vi "CheckAcqErrTlog.vi"(4 "error in":errorcluster) -> (0 "error out":errorcluster, 2 "Erreur":bool)   [LabVIEW 2010]
doc: "Ce Vi prend un tableau de donnée et convertit chaque donées selon la fonction spécifié par l'indicateur du même index dans la table de conversion."
uses:
  <userlib>/TLogger/AcqErrorGlobalTlog.vi
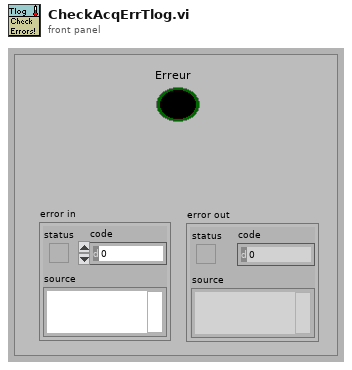
[diagram p1: front panel]
types:
  T1 = enum32{"Invalid", "Standard", "Closed", "Hidden", "Minimized", "Maximized"}
  T2 = enum32{"Bad", "Idle", "Run top level", "Running"}
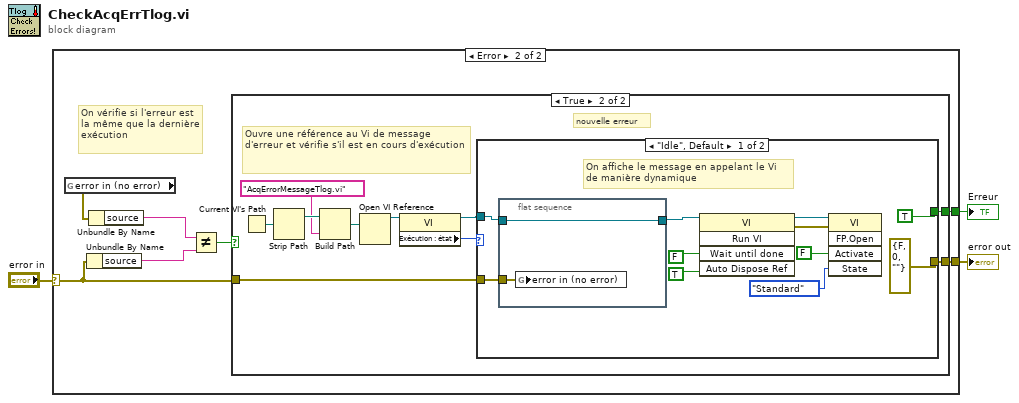
[diagram p0: block diagram]
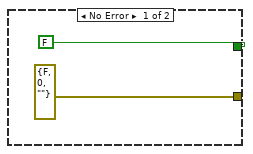
[diagram p2: hidden frame]
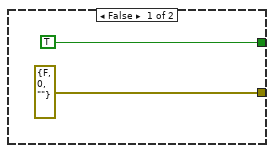
[diagram p3: hidden frame]
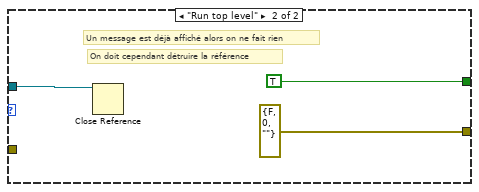
[diagram p4: hidden frame]
diagram:
  n1 = case shown="Error" "error in" {
    selector: "error in" -> [_ w10]
    tunnel: [errorcluster {"status"=FALSE, "code"=0, "source"=""} ("error out") w12] -> w2
    tunnel: [FALSE ("status") w11] -> w1
    frame No Error {
    }
    frame Error {
      # "On vérifie si l'erreur est la même que la dernière exécution"
      n2 = global read "AcqErrorGlobalTlog.vi" "error in (no error)"() -> (w9:errorcluster)
      n3 = Unbundle By Name(w10) -> ("source"=w8:string)
      n4 = Unbundle By Name(w9) -> ("source"=w7:string)
      n5 = Not Equal?(x=w7, y=w8) -> (x != y?=w6:bool)
      n6 = case shown="True" w6 {
        tunnel: w10 -> [_ w24]
        tunnel: [errorcluster {"status"=FALSE, "code"=0, "source"=""} ("error out") w23] -> w12
        tunnel: [TRUE ("status") w22] -> w11
        frame False {
        }
        frame True {
          # "nouvelle erreur"
          # "Ouvre une référence au Vi de message d'erreur et vérifie s'il est en cours d'exécution"
          n7 = Current VI's Path() -> (path=w21:path)
          n8 = Strip Path(path=w21) -> (stripped path=w20:path)  [unwired: 1 out]
          n9 = Build Path(base path=w20, name or relative path="AcqErrorMessageTlog.vi") -> (appended path=w18:path)
          n10 = Open VI Reference(vi path=w18) -> (vi reference=w17:refnum<vi>)  [unwired: 5 in, 1 out]
          n11 = property class="VI"(reference=w17) -> (reference out=w16:refnum<vi>, "Exécution : état"=w15:T2)  [unwired: 1 in, 1 out]
          n12 = case shown="\"Idle\", Default" w15 {
            tunnel: w24 -> [w31 _]
            tunnel: [errorcluster {"status"=FALSE, "code"=0, "source"=""} ("error out") errorcluster {"status"=FALSE, "code"=0, "source"=""} ("error out")] -> w23
            tunnel: [TRUE ("status") TRUE ("status")] -> w22
            tunnel: w16 -> [w30 w38]
            frame "Idle", Default {
              # "On affiche le message en appelant le Vi de manière dynamique"
              n13 = flat-sequence {
                tunnel: w31 -> [w37]
                tunnel: w30 -> [w36]
                tunnel: [w36] -> w29
                frame #0 {
                  n14 = global write "AcqErrorGlobalTlog.vi" "error in (no error)"(w37) -> ()
                }
              }
              n15 = invoke class="VI" method="Run VI"(reference=w29, "Wait until done"=FALSE, "Auto Dispose Ref"=TRUE) -> (reference out=w28:refnum<vi>, error out=w25:errorcluster)  [unwired: 2 in, 3 out]
              n16 = invoke class="VI" method="FP.Open"(reference=w28, error in=w25, "Activate"=FALSE, "State"=T1."Standard") -> ()  [unwired: 1 in, 5 out]
            }
            frame "Run top level" {
              # "On doit cependant détruire la référence"
              # "Un message est déjà affiché alors on ne fait rien"
              n17 = Close Reference(reference=w38) -> ()  [unwired: 1 in, 1 out]
            }
          }
        }
      }
    }
  }
  "error out" <- w2
  "Erreur" <- w1
